vi "input.vi"(9 "Z":dbl, 10 "Y":dbl, 11 "X":dbl) -> (3 "yo":dbl[](array[numeric]))   [LabVIEW 2015]
uses:
  <vilib>/imath/engines/lvmath2/RunTimeEngine/ArithmeticOperatorToken/NIMS_ArithmeticOperator_multmx(M,CV)-internal.vi
  <instcachedir>/0/NIMS_ArithmeticOperator_multmx(M,CV)-internal_4015640DB52447B392A036248F93EE7C.lvgen/NIMS_ArithmeticOperator_multmx(M,CV)-internal_4015640DB52447B392A036248F93EE7C_001.vi
  <vilib>/imathl/engines/lvmath/Functions/Error Handling/Create Error.vi
  <vilib>/imath/engines/lvmath2/RunTimeEngine/NodeEndStatement/NIMS_NodeEndStatement_Output.vi
  <instcachedir>/0/NIMS_NodeEndStatement_Output_53EC0D466D134D7ABD903AC30B43404B.lvgen/NIMS_NodeEndStatement_Output_53EC0D466D134D7ABD903AC30B43404B_005.vi
  <vilib>/imath/engines/lvmath2/RunTimeEngine/ErrorHandling/NIMS_Finalize Error.vi
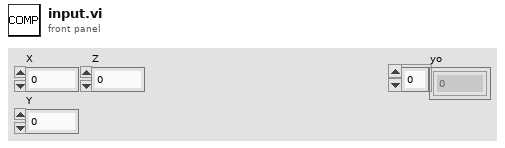
[diagram p1: front panel]
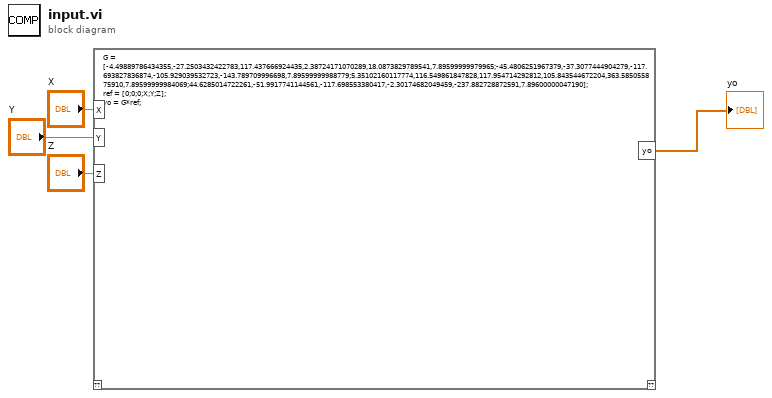
[diagram p0: block diagram]
diagram:
  n1 = mathscript code="G = [-4.49889786434355,-27.2503432422783,117.437666924435,2.38724171070289,18.0873829789541,7.89599999979965;-45.4806251967379,-37.3077444904279,-117.693827836874,-105.929039532723,-143.789709996698,7.89599999988779;5.35102160117774,116.549861847828,117.954714292812,105.843544672204,363.585055875910,7.89599999984069;44.6285014722261,-51.9917741144561,-117.698553380417,-2.30174682049459,-237.882728872591,7.89600000047190];\nref = [0;0;0;X;Y;Z];\nyo = G*ref;"("X"="X", "Y"="Y", "Z"="Z") -> ("yo"=→"yo":dbl[])  [unwired: 1 in, 1 out]
